vi "Connect to Error Handles.vi"(8 "error in":errorcluster, 9 "Timeout (ms)":u16, 11 "Async in":refnum<class "VS Inline Async API.lvclass">) -> (0 "error out":errorcluster, 3 "Async out":refnum<class "VS Inline Async API.lvclass">)   [LabVIEW 2015, in "VS Inline Async API.lvlib" / "VS Inline Async API.lvclass"]
uses:
  VS Inline Async API.lvclass
  VS Inline Async API.lvclass/VS Inline Async API.ctl
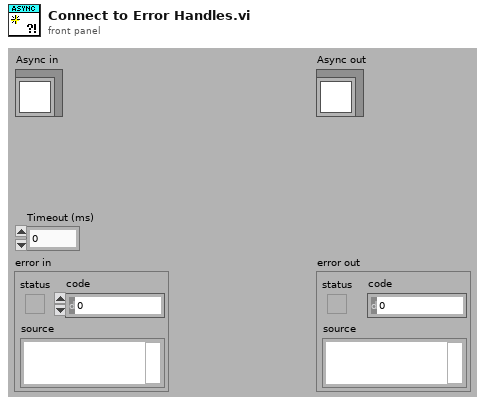
[diagram p1: front panel]
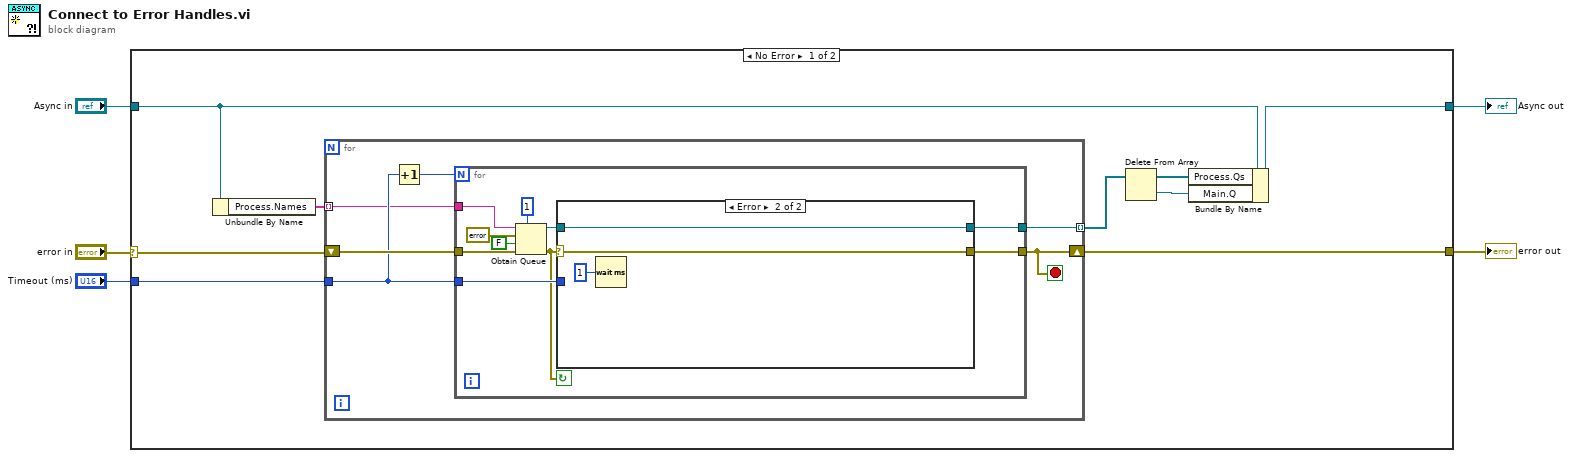
[diagram p0: block diagram]
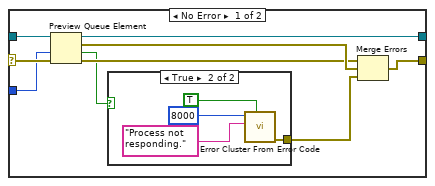
[diagram p2: hidden frame]
diagram:
  n1 = case shown="No Error" "error in" {
    selector: "error in" -> [w13 w48]
    tunnel: [w9 w48] -> w5
    tunnel: "Timeout (ms)" -> [w14 _]
    tunnel: "Async in" -> [w11 w47]
    tunnel: [w12 w47] -> w1
    frame No Error {
      n2 = Unbundle By Name(w11) -> ("Process.Names"=w10:string[])
      n3 = for {
        shift-right: [w16] -> w9
        shift-left: w13 -> [w20]
        tunnel: [w19] -> w8 mode=indexing
        tunnel: w14 -> [w17]
        tunnel: w10 -> [w15] mode=indexing
        stop <- w16 stop-if-true
        n4 = Increment(x=w17) -> (x+1=w18:u16)
        n5 = for {
          N: w18 -> [_]
          tunnel: [w26] -> w19
          tunnel: w17 -> [w24]
          tunnel: w20 -> [w28]
          tunnel: [w23] -> w16
          tunnel: w15 -> [w21]
          stop <- w22 continue-if-true
          n6 = Obtain Queue(max queue size (-1, unlimited)=1, name (unnamed)=w21, element data type=errorcluster {"status"=FALSE, "code"=0, "source"=""} ("error out"), create if not found? (T)=FALSE, error in (no error)=w28) -> (queue out=w25:refnum<queue>, error out=w22:errorcluster)  [unwired: 1 out]
          n7 = case shown="Error" w22 {
            selector: w22 -> [w37 w46]
            tunnel: [w33 w46] -> w23
            tunnel: [w38 w45] -> w26
            tunnel: w25 -> [w39 w45]
            tunnel: w24 -> [w36 _]
            frame No Error {
              n8 = Preview Queue Element(queue=w39, timeout in ms (-1)=w36, error in (no error)=w37) -> (queue out=w38:refnum<queue>, element=w35:errorcluster, timed out?=w31:bool, error out=w34:errorcluster)
              n9 = case shown="True" w31 {
                tunnel: [_ w43] -> w32
                frame False {
                }
                frame True {
                  n10 = call <vilib>:"Error Cluster From Error Code.vi"("show call chain? (False)"=TRUE, "error message (\"\")"="Process not responding." ("source"), "error code (0)"=8000) -> ("error out"=w43:errorcluster)  [unwired: 6 in]
                }
              }
              n11 = Merge Errors(w34, w35, w32) -> (w33:errorcluster)
            }
            frame Error {
              n12 = Wait (ms)(milliseconds to wait=u32 1) -> ()  [unwired: 1 out]
            }
          }
        }
      }
      n13 = Delete From Array(array=w8) -> (deleted portion=w6:refnum<queue>, array with subset deleted=w7:refnum<queue>[])  [unwired: 2 in]
      n14 = Bundle By Name(cluster=w11, "Process.Qs"=w7, "Main.Q"=w6) -> (w12:refnum<class "VS Inline Async API.lvclass">)
    }
    frame Error {
    }
  }
  "error out" <- w5
  "Async out" <- w1
